vi "Kontrol Y.vi"(0 "denge degeri":dbl, 5 "İterasyon Denge":dbl, 7 "Denge Kosulu y1_y2":dbl[][](array[numeric]), 9 "Manuel/Otomatik":enum16{"Manuel", "Otomatik"}(ring)=enum."Otomatik", 11 "frekans index":dbl) -> (4 "Denge Seçimi":u8=4 min=1 max=5, 6 "New İterasyon Denge":dbl, 8 "Iterasyon Count Successful":dbl, 15 "Start Denge Y":bool)   [LabVIEW 2014]
panel:
  in  "GPIB In":refnum<visa-resource-name>="GPIB0::8::INSTR"
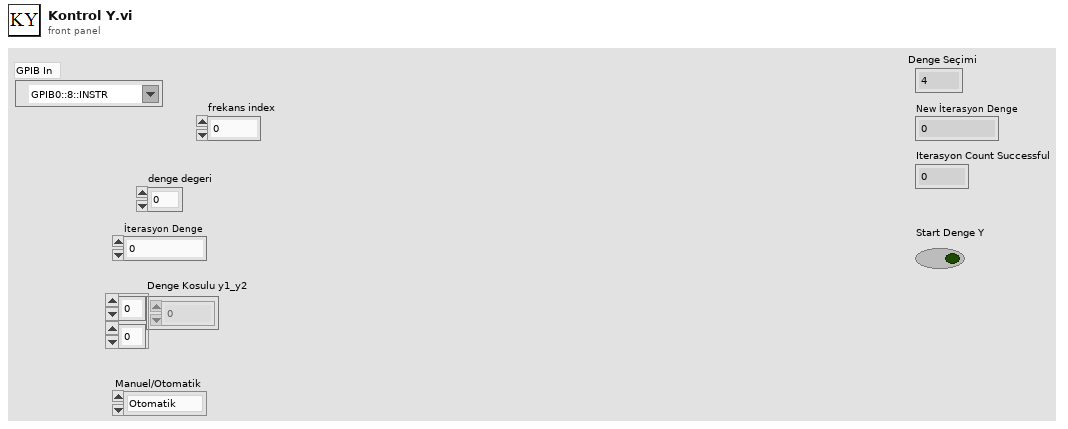
[diagram p1: front panel]
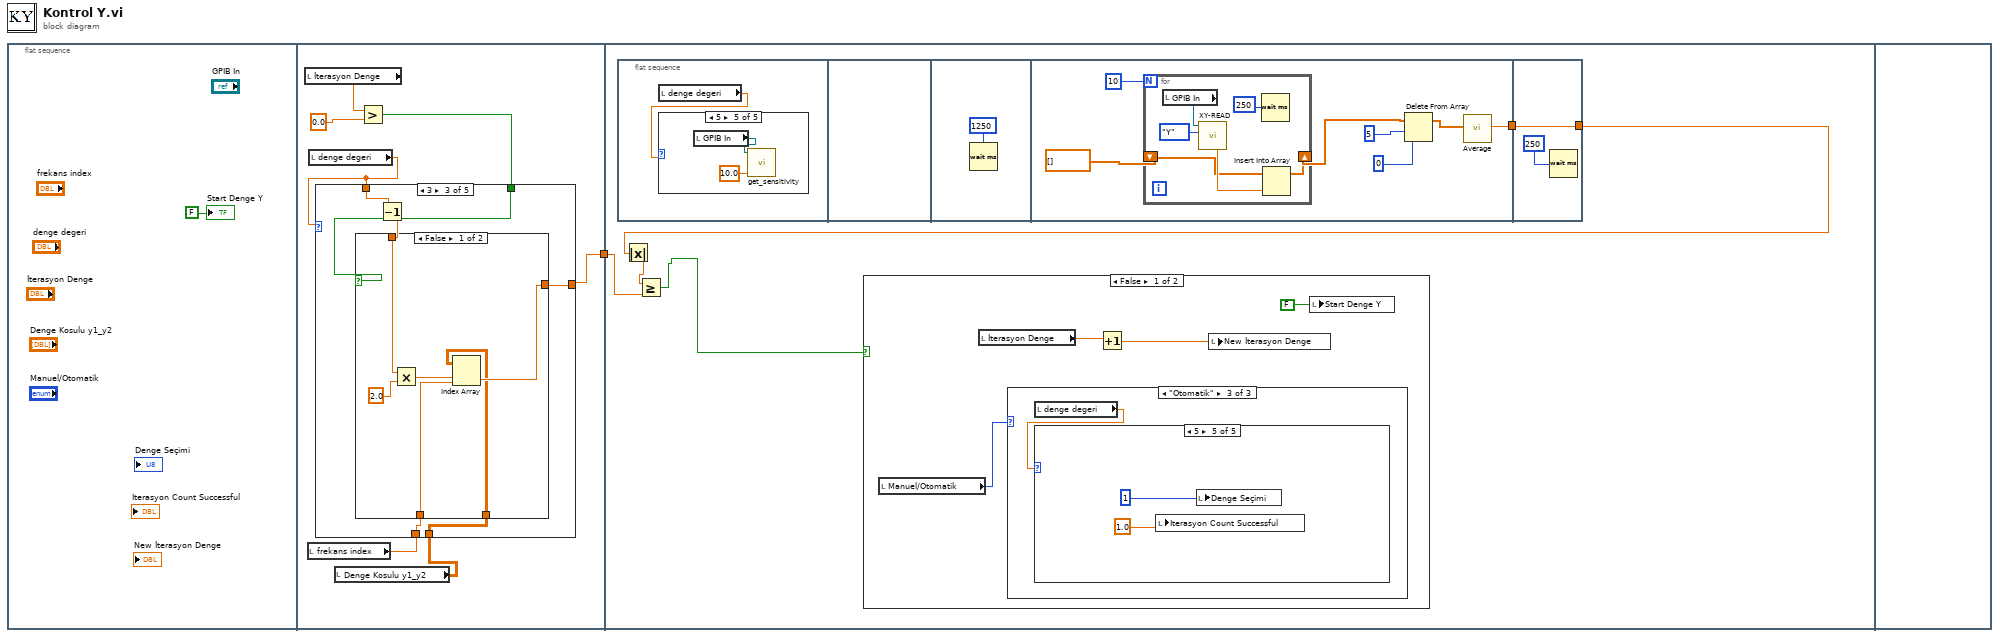
[diagram p0: block diagram]
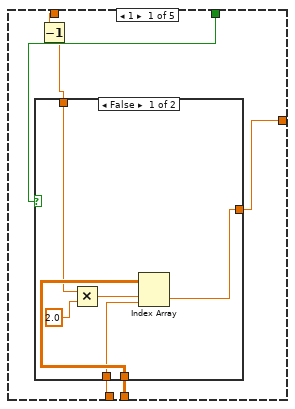
[diagram p2: hidden frame]
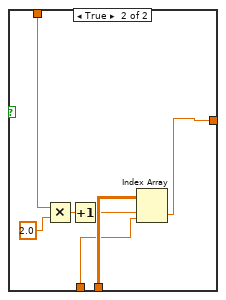
[diagram p3: hidden frame]
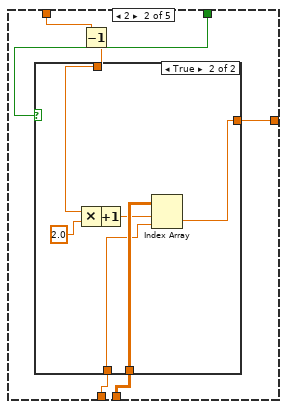
[diagram p4: hidden frame]
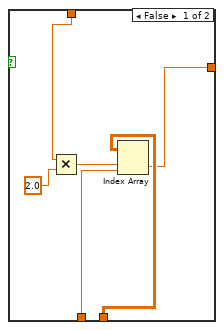
[diagram p5: hidden frame]
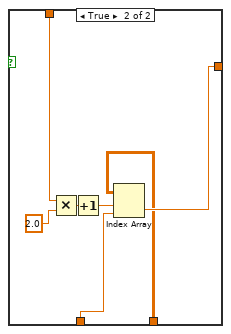
[diagram p6: hidden frame]
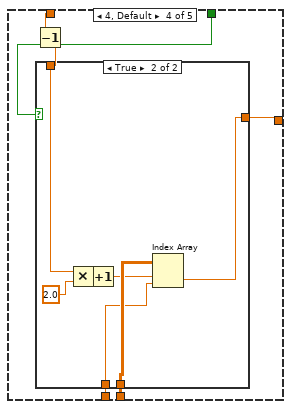
[diagram p7: hidden frame]
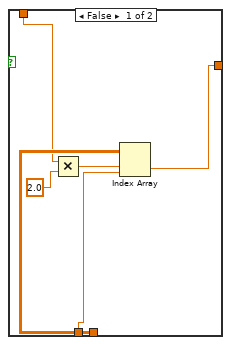
[diagram p8: hidden frame]
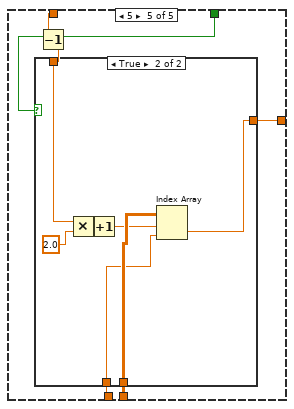
[diagram p9: hidden frame]
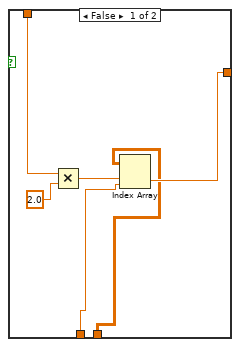
[diagram p10: hidden frame]
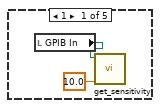
[diagram p11: hidden frame]
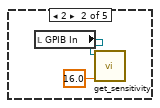
[diagram p12: hidden frame]
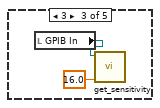
[diagram p13: hidden frame]
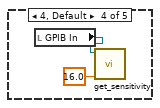
[diagram p14: hidden frame]
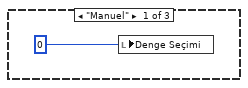
[diagram p15: hidden frame]
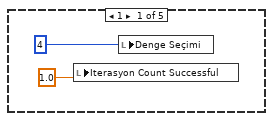
[diagram p17: hidden frame]
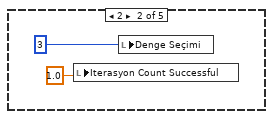
[diagram p18: hidden frame]
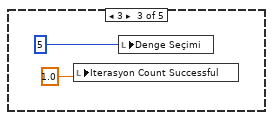
[diagram p19: hidden frame]
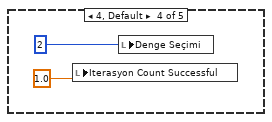
[diagram p20: hidden frame]
diagram:
  n1 = flat-sequence {
    tunnel: [w7] -> w1
    tunnel: w1 -> [w108]
    frame #0 {
      "Start Denge Y" <- FALSE ("Start Denge")
    }
    frame #1 {
      n2 = local read "İterasyon Denge"() -> (w6:dbl)
      n3 = local read "frekans index"() -> (w3:dbl)
      n4 = local read "denge degeri"() -> (w5:dbl)
      n5 = local read "Denge Kosulu y1_y2"() -> (w4:dbl[][])
      n6 = Greater?(x=w6, y=0.0) -> (0:w8:bool)
      n7 = case shown="3" w5 {
        tunnel: w8 -> [w15 w34 w53 w72 w91]
        tunnel: [w14 w33 w52 w71 w90] -> w7
        tunnel: w5 -> [w13 w31 w51 w69 w88]
        tunnel: w4 -> [w12 w32 w50 w70 w89]
        tunnel: w3 -> [w10 w29 w48 w67 w86]
        frame 1 {
          n8 = Decrement(x=w13) -> (x-1=w11:dbl)
          n9 = case shown="False" w15 {
            tunnel: [w19 w25] -> w14
            tunnel: w11 -> [w18 w26]
            tunnel: w12 -> [w20 w24]
            tunnel: w10 -> [w16 w22]
            frame False {
              n10 = Multiply(x=w18, y=2.0) -> (x*y=w17:dbl)
              n11 = Index Array(array=w20, index (row)=w17, index (col)=w16) -> (element=w19:dbl)
            }
            frame True {
              n12 = Multiply(x=w26, y=2.0) -> (x*y=w27:dbl)
              n13 = Increment(x=w27) -> (x+1=w23:dbl)
              n14 = Index Array(array=w24, index (row)=w23, index (col)=w22) -> (element=w25:dbl)
            }
          }
        }
        frame 2 {
          n15 = Decrement(x=w31) -> (x-1=w30:dbl)
          n16 = case shown="True" w34 {
            tunnel: [w37 w45] -> w33
            tunnel: w32 -> [w38 w44]
            tunnel: w30 -> [w39 w43]
            tunnel: w29 -> [w35 w41]
            frame False {
              n17 = Multiply(x=w39, y=2.0) -> (x*y=w36:dbl)
              n18 = Index Array(array=w38, index (row)=w36, index (col)=w35) -> (element=w37:dbl)
            }
            frame True {
              n19 = Multiply(x=w43, y=2.0) -> (x*y=w46:dbl)
              n20 = Increment(x=w46) -> (x+1=w42:dbl)
              n21 = Index Array(array=w44, index (row)=w42, index (col)=w41) -> (element=w45:dbl)
            }
          }
        }
        frame 3 {
          n22 = Decrement(x=w51) -> (x-1=w49:dbl)
          n23 = case shown="False" w53 {
            tunnel: [w58 w64] -> w52
            tunnel: w49 -> [w57 w63]
            tunnel: w50 -> [w56 w62]
            tunnel: w48 -> [w54 w60]
            frame False {
              n24 = Multiply(x=w57, y=2.0) -> (x*y=w55:dbl)
              n25 = Index Array(array=w56, index (row)=w55, index (col)=w54) -> (element=w58:dbl)
            }
            frame True {
              n26 = Multiply(x=w63, y=2.0) -> (x*y=w65:dbl)
              n27 = Increment(x=w65) -> (x+1=w61:dbl)
              n28 = Index Array(array=w62, index (row)=w61, index (col)=w60) -> (element=w64:dbl)
            }
          }
        }
        frame 4, Default {
          n29 = Decrement(x=w69) -> (x-1=w68:dbl)
          n30 = case shown="True" w72 {
            tunnel: [w77 w83] -> w71
            tunnel: w70 -> [w76 w82]
            tunnel: w68 -> [w75 w81]
            tunnel: w67 -> [w73 w79]
            frame False {
              n31 = Multiply(x=w75, y=2.0) -> (x*y=w74:dbl)
              n32 = Index Array(array=w76, index (row)=w74, index (col)=w73) -> (element=w77:dbl)
            }
            frame True {
              n33 = Multiply(x=w81, y=2.0) -> (x*y=w84:dbl)
              n34 = Increment(x=w84) -> (x+1=w80:dbl)
              n35 = Index Array(array=w82, index (row)=w80, index (col)=w79) -> (element=w83:dbl)
            }
          }
        }
        frame 5 {
          n36 = Decrement(x=w88) -> (x-1=w87:dbl)
          n37 = case shown="True" w91 {
            tunnel: [w96 w102] -> w90
            tunnel: w89 -> [w95 w101]
            tunnel: w87 -> [w94 w100]
            tunnel: w86 -> [w92 w98]
            frame False {
              n38 = Multiply(x=w94, y=2.0) -> (x*y=w93:dbl)
              n39 = Index Array(array=w95, index (row)=w93, index (col)=w92) -> (element=w96:dbl)
            }
            frame True {
              n40 = Multiply(x=w100, y=2.0) -> (x*y=w103:dbl)
              n41 = Increment(x=w103) -> (x+1=w99:dbl)
              n42 = Index Array(array=w101, index (row)=w99, index (col)=w98) -> (element=w102:dbl)
            }
          }
        }
      }
    }
    frame #2 {
      n43 = flat-sequence {
        tunnel: [w122] -> w106
        tunnel: [w135] -> w105
        tunnel: w106 -> [w135]
        frame #0 {
          n44 = local read "denge degeri"() -> (w110:dbl)
          n45 = case shown="5" w110 {
            frame 1 {
              n46 = local read "GPIB In"() -> (w111:refnum<visa-resource-name>)
              n47 = call "get_sensitivity.vi"("input 1"=10.0, "SR850 GPIB In"=w111) -> ()  [unwired: 8 in, 2 out]
            }
            frame 2 {
              n48 = local read "GPIB In"() -> (w113:refnum<visa-resource-name>)
              n49 = call "get_sensitivity.vi"("input 1"=16.0, "SR850 GPIB In"=w113) -> ()  [unwired: 8 in, 2 out]
            }
            frame 3 {
              n50 = local read "GPIB In"() -> (w115:refnum<visa-resource-name>)
              n51 = call "get_sensitivity.vi"("input 1"=16.0, "SR850 GPIB In"=w115) -> ()  [unwired: 8 in, 2 out]
            }
            frame 4, Default {
              n52 = local read "GPIB In"() -> (w117:refnum<visa-resource-name>)
              n53 = call "get_sensitivity.vi"("input 1"=16.0, "SR850 GPIB In"=w117) -> ()  [unwired: 8 in, 2 out]
            }
            frame 5 {
              n54 = local read "GPIB In"() -> (w119:refnum<visa-resource-name>)
              n55 = call "get_sensitivity.vi"("input 1"=10.0, "SR850 GPIB In"=w119) -> ()  [unwired: 8 in, 2 out]
            }
          }
        }
        frame #1 {
        }
        frame #2 {
          n56 = Wait (ms)(milliseconds to wait=u32 1250) -> ()  [unwired: 1 out]
        }
        frame #3 {
          n57 = for {
            N: 10 -> [_]
            shift-right: [w131] -> w126
            shift-left: dbl[] [] -> [w130]
            n58 = local read "GPIB In"() -> (w134:refnum<visa-resource-name>)
            n59 = call "XY-READ.vi"("X/Y ?"=enum16{"X", "Y"}."Y" ("Enum"), "SR850 GPIB IN"=w134) -> ("SR850_Reading"=w132:dbl)  [unwired: 7 in, 2 out]
            n60 = Wait (ms)(milliseconds to wait=u32 250) -> ()  [unwired: 1 out]
            n61 = Insert Into Array(array=w130, new element=w132) -> (w131:dbl[])  [unwired: 1 in]
          }
          n62 = Delete From Array(array=w126, length=5, index=0) -> (array with subset deleted=w125:dbl[])  [unwired: 1 out]
          n63 = call "Average.vi"("Array"=w125) -> ("Average"=w122:dbl)  [unwired: 9 in, 1 out]
        }
        frame #4 {
          n64 = Wait (ms)(milliseconds to wait=u32 250) -> ()  [unwired: 1 out]
        }
      }
      n65 = Absolute Value(x=w105) -> (abs(x)=w109:dbl)
      n66 = Greater Or Equal?(x=w109, y=w108) -> (x >= y?=w107:bool)
      n67 = case shown="False" w107 {
        frame False {
          n68 = local read "Manuel/Otomatik"() -> (w137:enum16{"Manuel", "Otomatik"})
          n69 = local read "İterasyon Denge"() -> (w139:dbl)
          n70 = case shown="\"Otomatik\"" w137 {
            frame "Manuel" {
              n71 = local write "Denge Seçimi"(u32 0 ("Çalıştırmak istediğiniz Programı Seçin")) -> ()
            }
            frame Default {
            }
            frame "Otomatik" {
              n72 = local read "denge degeri"() -> (w142:dbl)
              n73 = case shown="5" w142 {
                frame 1 {
                  n74 = local write "Iterasyon Count Successful"(1.0 ("Iterasyon Successful")) -> ()
                  n75 = local write "Denge Seçimi"(u32 4 ("Çalıştırmak istediğiniz Programı Seçin")) -> ()
                }
                frame 2 {
                  n76 = local write "Iterasyon Count Successful"(1.0 ("Iterasyon Successful")) -> ()
                  n77 = local write "Denge Seçimi"(u32 3 ("Çalıştırmak istediğiniz Programı Seçin")) -> ()
                }
                frame 3 {
                  n78 = local write "Iterasyon Count Successful"(1.0 ("Iterasyon Successful")) -> ()
                  n79 = local write "Denge Seçimi"(u32 5 ("Çalıştırmak istediğiniz Programı Seçin")) -> ()
                }
                frame 4, Default {
                  n80 = local write "Iterasyon Count Successful"(1.0 ("Iterasyon Successful")) -> ()
                  n81 = local write "Denge Seçimi"(u32 2 ("Çalıştırmak istediğiniz Programı Seçin")) -> ()
                }
                frame 5 {
                  n82 = local write "Iterasyon Count Successful"(1.0 ("Iterasyon Successful")) -> ()
                  n83 = local write "Denge Seçimi"(u32 1 ("Çalıştırmak istediğiniz Programı Seçin")) -> ()
                }
              }
            }
          }
          n84 = Increment(x=w139) -> (x+1=w138:dbl)
          n85 = local write "New İterasyon Denge"(w138) -> ()
          n86 = local write "Start Denge Y"(FALSE ("Start Mod")) -> ()
        }
        frame True {
          n87 = local write "Start Denge Y"(TRUE ("Start Mod")) -> ()
        }
      }
    }
    frame #3 {
    }
  }
